vi "Add Sheet.vi"(8 "error in":errorcluster, 10 "SheetName":string, 11 "SpreadsheetDocument in":refnum<k24>) -> (0 "error out":errorcluster, 3 "SpreadsheetDocument out":refnum<k24>)   [LabVIEW 2021, in "Open Xml.lvlib"]
uses:
  Open Xml.lvlib
  D:/git/Open-Xml-LabVIEW/dll/DocumentFormat.OpenXml.dll
  dll/DocumentFormat.OpenXml.dll
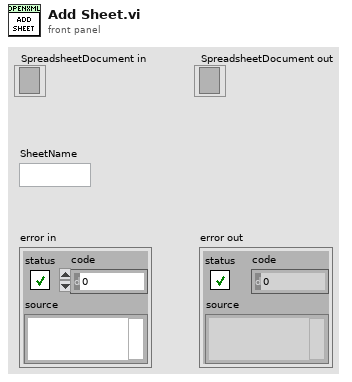
[diagram p1: front panel]
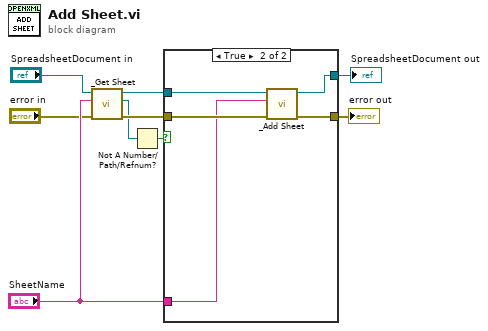
[diagram p0: block diagram]
diagram:
  n1 = call "_Get Sheet.vi"("error in"="error in", "SheetName"="SheetName", "SpreadsheetDocument in"="SpreadsheetDocument in") -> ("error out"=w3:errorcluster, "Sheet"=w1:refnum<k24>, "SpreadsheetDocument out"=w2:refnum<k24>)  [unwired: 6 in]
  n2 = Not A Number/Path/Refnum?(number/path/refnum=w1) -> (NaN/Path/Refnum?=w4:bool)
  n3 = case shown="True" w4 {
    tunnel: [w10 w13] -> w9
    tunnel: [w11 w12] -> w8
    tunnel: "SheetName" -> [_ w14]
    tunnel: w3 -> [w11 w16]
    tunnel: w2 -> [w10 w15]
    frame False {
    }
    frame True {
      n4 = call "_Add Sheet.vi"("error in"=w16, "SheetName"=w14, "SpreadsheetDocument in"=w15) -> ("error out"=w12:errorcluster, "SpreadsheetDocument out"=w13:refnum<k24>)  [unwired: 7 in]
    }
  }
  "error out" <- w8
  "SpreadsheetDocument out" <- w9
